vi "Actor Core.vi"(8 "error in":errorcluster, 11 "Universal Power Meter in":refnum<class "Universal Power Meter.lvclass">) -> (0 "error out":errorcluster, 3 "Actor out":refnum<class "Actor.lvclass">)   [LabVIEW 2012]
doc: "(<B>Filename</B>: Actor Framework.lvlib:Actor.lvclass:Actor Core.vi)\n\nReceives messages to the actor, reacts to them, and initiates any error handling that may shut the actor down.\n\nDescendant classes may override this VI to append parallel tasks for the actor to complete while it handles messages. Overrides use the Call Parent Method node."
uses:
  Universal Power Meter.lvclass
  <vilib>/ActorFramework/Actor/Actor.lvclass
panel:
  out "Number of Cards":dbl
  out "Power Meter Visa":refnum<visa-resource-name>
  out "Instrument ID":string
  out "ID cluster.Model":string
  out "Manufacturer":string
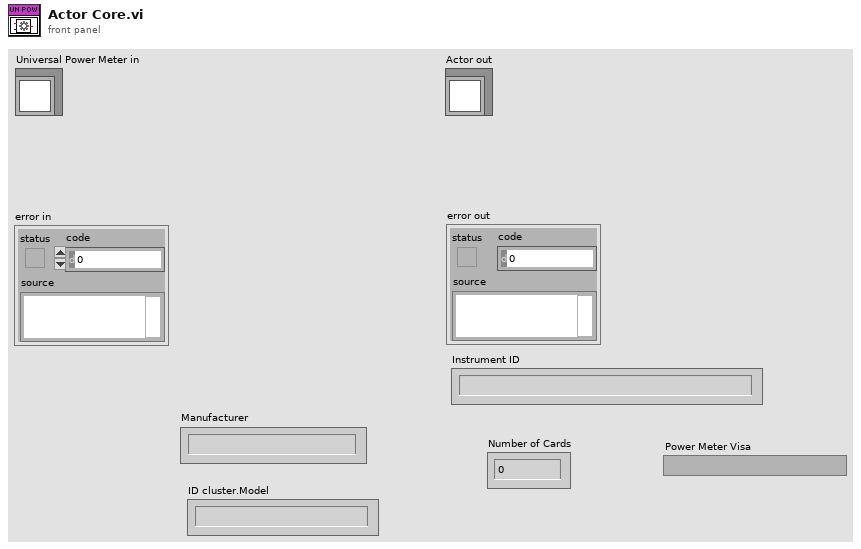
[diagram p1: front panel]
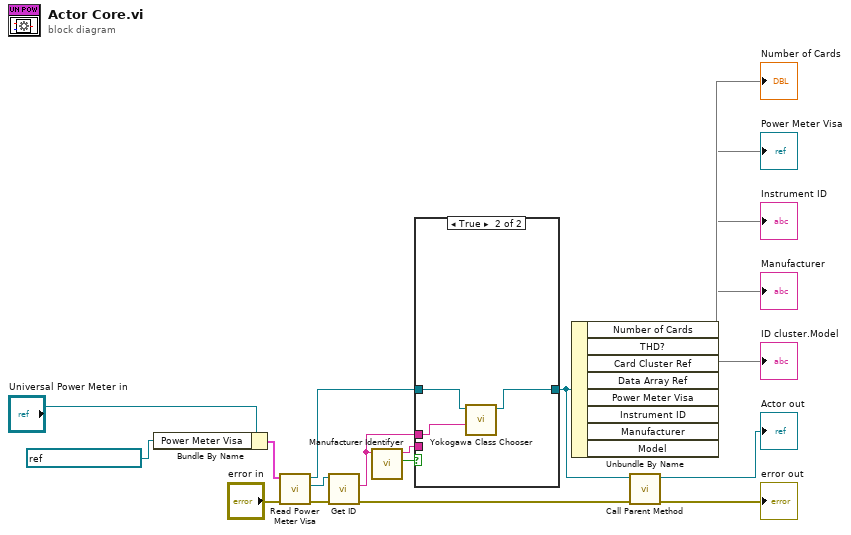
[diagram p0: block diagram]
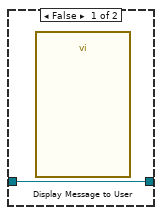
[diagram p2: hidden frame]
diagram:
  n1 = Bundle By Name(cluster="Universal Power Meter in", "Power Meter Visa"=refnum<visa-resource-name> "GPIB0::30::INSTR") -> (w2:cluster{})
  n2 = call "Read Power Meter Visa.vi"("error in (no error)"="error in", "Universal Power Meter in"=w2) -> ("error out"=w16:errorcluster, "Power Meter Visa"=w17:refnum<visa-resource-name>, "Universal Power Meter out"=w11:refnum<class "Universal Power Meter.lvclass">)  [unwired: 7 in]
  n3 = call "Get ID.vi"("error in (no error)"=w16, "VISA resource name"=w17) -> ("error out"=w4:errorcluster, "read buffer"=w12:string)  [unwired: 7 in, 1 out]
  n4 = call "Manufacturer Identifyer.vi"("read buffer"=w12) -> ("Boolean"=w14:bool, "string"=w13:string)  [unwired: 9 in]
  n5 = case shown="True" w14 {
    tunnel: w13 -> [_ _]
    tunnel: w12 -> [_ w23]
    tunnel: w11 -> [w20 w22]
    tunnel: [w20 w21] -> w10
    frame False {
      n6 = call "Display Message to User"() -> ()  [unwired: 10 in, 2 out]
    }
    frame True {
      n7 = call-dynamic "Yokogawa Class Chooser.vi"("Incoming ID"=w23, "Universal Power Meter.lvlib:Universal Power Meter.lvclass"=w22) -> ("Class out"=w21:refnum<class "Universal Power Meter.lvclass">)  [unwired: 9 in]
    }
  }
  n8 = Unbundle By Name(w10) -> ("Number of Cards"=→"Number of Cards", "Power Meter Visa"=→"Power Meter Visa", "Instrument ID"=→"Instrument ID", "Manufacturer"=→"Manufacturer", "Model"=→"ID cluster.Model")  [unwired: 3 out]
  n9 = call-parent "Call Parent Method"("error in"=w4, "Actor in"=w10) -> ("error out"=→"error out":errorcluster, "Actor out"=→"Actor out":refnum<class "Actor.lvclass">)  [unwired: 8 in]
